vi "setAngle_00.vi"(1 "error in (no error)":errorcluster, 2 "Angle (deg)":dbl) -> (0 "error out":errorcluster)   [LabVIEW 2011]
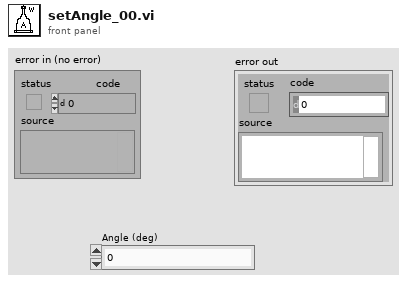
[diagram p1: front panel]
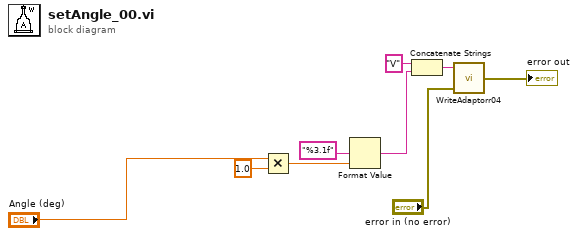
[diagram p0: block diagram]
diagram:
  n1 = Multiply(x="Angle (deg)", y=1.0) -> (x*y=w8:dbl)
  n2 = Format Value(format string="%3.1f", value (0)=w8) -> (output string=w9:string)  [unwired: 1 in]
  n3 = Concatenate Strings("V" ("string"), w9) -> (w6:string)
  n4 = call "WriteAdaptorr04.vi"("error in (no error)"="error in (no error)", "string to write"=w6) -> ("error out"=→"error out":errorcluster)  [unwired: 1 in]
